vi "PointStep_Control.vi"(8 "error in (no error)":errorcluster, 9 "Temp and Field Range in":T1, 10 "ACK Q":refnum<queue>, 11 "Queue in":refnum<queue>) -> (0 "error out":errorcluster, 2 "Temp and Field Range out":T1, 3 "Queue out":refnum<queue>)   [LabVIEW 2025]
uses:
  CTLS/Sweeper.ctl
  CTLS/ACK.ctl
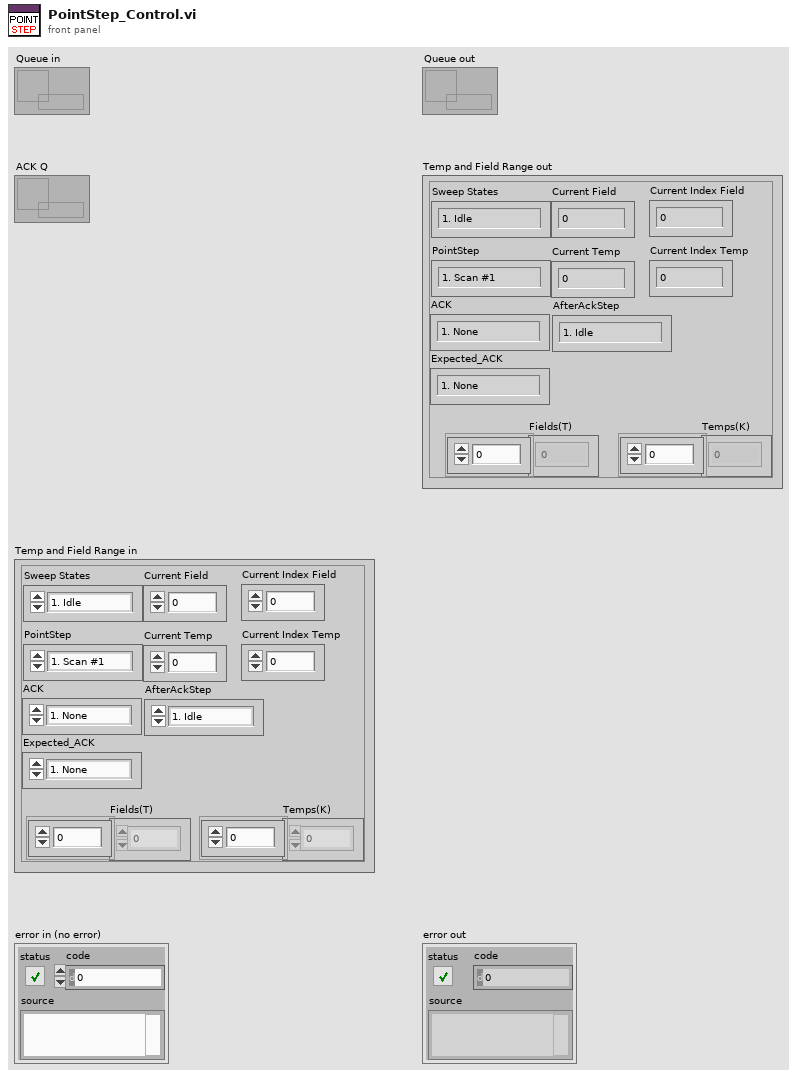
[diagram p1: front panel]
types:
  T1 = typedef "Sweeper.ctl" = cluster{"Temps(K)":dbl[], "Fields(T)":dbl[], "Sweep States":enum16{"1. Idle", "2. Start", "3. Apply_Config", "4. Run_Point_Step", "5. Wait ACK", "6. Next Field", "6. Next Temp", "8. Stop"}, "PointStep":enum16{"1. Scan #1", "2. Drift Correct (SF) #1", "3. Drift Correct (BS) #1", "4. Bias", "5. Scan #2", "6. Drift Correct (SF) #2", "7. Drift Correct (BS) #2", "8. Done"}, "Current Field":dbl, "Current Temp":dbl, "Expected_ACK":enum16{"1. None", "2. TempStable", "3. FieldStable", "4. ConfigApplied", "5. ScanDone", "6. BiasDone", "7. DriftDone (SF)", "8. DrifDone (BS)", "9. Done"}, "ACK":enum16{"1. None", "2. TempStable", "3. FieldStable", "4. ConfigApplied", "5. ScanDone", "6. BiasDone", "7. DriftDone (SF)", "8. DrifDone (BS)", "9. Done"}, "AfterAckStep":enum16{"1. Idle", "2. Start", "3. Apply_Config", "4. Run_Point_Step", "5. Wait ACK", "6. Next Field", "6. Next Temp", "8. Stop"}, "Current Index Field":i32, "Current Index Temp":i32}
  T2 = typedef "ACK.ctl" = cluster{"ACK":enum16{"1. None", "2. TempStable", "3. FieldStable", "4. ConfigApplied", "5. ScanDone", "6. BiasDone", "7. DriftDone (SF)", "8. DrifDone (BS)"}}
  T3 = enum16{"1. None", "2. TempStable", "3. FieldStable", "4. ConfigApplied", "5. ScanDone", "6. BiasDone", "7. DriftDone (SF)", "8. DrifDone (BS)", "9. Done"}
  T4 = enum16{"1. None", "2. TempStable", "3. FieldStable", "4. ConfigApplied", "5. ScanDone", "6. BiasDone", "7. DriftDone (SF)", "8. DrifDone (BS)"}
  T5 = enum16{"1. Idle", "2. Start", "3. Apply_Config", "4. Run_Point_Step", "5. Wait ACK", "6. Next Field", "6. Next Temp", "8. Stop"}
  T6 = enum16{"1. Scan #1", "2. Drift Correct (SF) #1", "3. Drift Correct (BS) #1", "4. Bias", "5. Scan #2", "6. Drift Correct (SF) #2", "7. Drift Correct (BS) #2", "8. Done"}
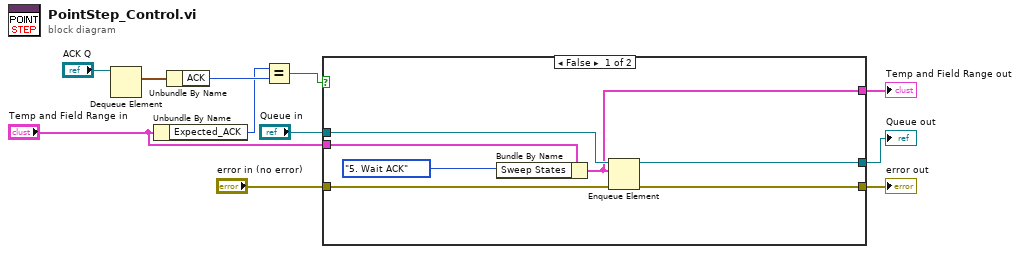
[diagram p0: block diagram]
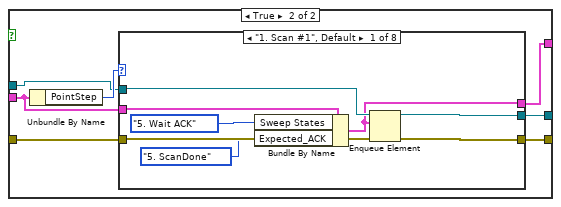
[diagram p2: hidden frame]
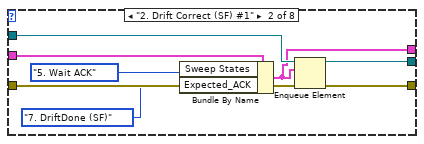
[diagram p3: hidden frame]
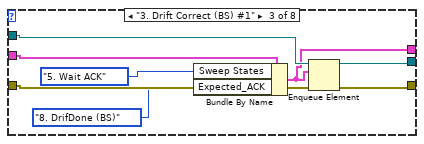
[diagram p4: hidden frame]
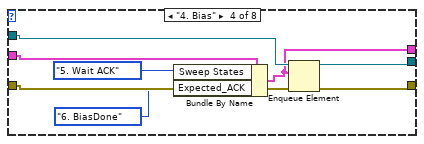
[diagram p5: hidden frame]
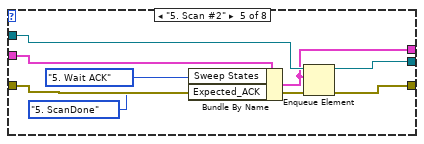
[diagram p6: hidden frame]
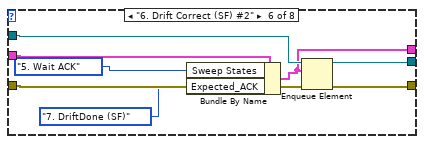
[diagram p7: hidden frame]
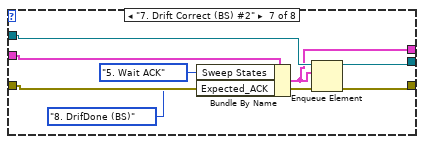
[diagram p8: hidden frame]
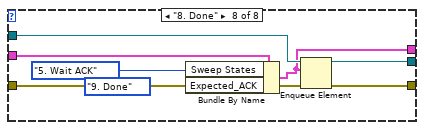
[diagram p9: hidden frame]
diagram:
  n1 = Dequeue Element(queue="ACK Q") -> (element=w2:T2)  [unwired: 2 in, 3 out]
  n2 = Unbundle By Name("Temp and Field Range in") -> ("Expected_ACK"=w3:T3)
  n3 = Unbundle By Name(w2) -> ("ACK"=w4:T4)
  n4 = Equal?(x=w3, y=w4) -> (x = y?=w5:bool)
  n5 = case shown="False" w5 {
    tunnel: "Queue in" -> [w18 w24]
    tunnel: "Temp and Field Range in" -> [w17 w23]
    tunnel: [w16 w22] -> w8
    tunnel: [w15 w21] -> w9
    tunnel: "error in (no error)" -> [w14 w20]
    tunnel: [w13 w19] -> w11
    frame False {
      n6 = Bundle By Name(cluster=w17, "Sweep States"=T5."5. Wait ACK") -> (w13:T1)
      n7 = Enqueue Element(queue=w18, element=w13, error in (no error)=w14) -> (queue out=w16:refnum<queue>, error out=w15:errorcluster)  [unwired: 1 in, 1 out]
    }
    frame True {
      n8 = Unbundle By Name(w23) -> ("PointStep"=w25:T6)
      n9 = case shown="\"1. Scan #1\", Default" w25 {
        tunnel: w24 -> [w33 w41 w49 w57 w65 w73 w81 w89]
        tunnel: w23 -> [w32 w40 w48 w56 w64 w72 w80 w88]
        tunnel: [w31 w38 w46 w54 w62 w70 w78 w86] -> w22
        tunnel: [w30 w37 w45 w53 w61 w68 w77 w85] -> w21
        tunnel: w20 -> [w29 w39 w47 w55 w63 w71 w79 w87]
        tunnel: [w28 w36 w44 w52 w60 w69 w76 w84] -> w19
        frame "1. Scan #1", Default {
          n10 = Bundle By Name(cluster=w32, "Sweep States"=T5."5. Wait ACK", "Expected_ACK"=T3."5. ScanDone") -> (w28:T1)
          n11 = Enqueue Element(queue=w33, element=w28, error in (no error)=w29) -> (queue out=w31:refnum<queue>, error out=w30:errorcluster)  [unwired: 1 in, 1 out]
        }
        frame "2. Drift Correct (SF) #1" {
          n12 = Bundle By Name(cluster=w40, "Sweep States"=T5."5. Wait ACK", "Expected_ACK"=T3."7. DriftDone (SF)") -> (w36:T1)
          n13 = Enqueue Element(queue=w41, element=w36, error in (no error)=w39) -> (queue out=w38:refnum<queue>, error out=w37:errorcluster)  [unwired: 1 in, 1 out]
        }
        frame "3. Drift Correct (BS) #1" {
          n14 = Bundle By Name(cluster=w48, "Sweep States"=T5."5. Wait ACK", "Expected_ACK"=T3."8. DrifDone (BS)") -> (w44:T1)
          n15 = Enqueue Element(queue=w49, element=w44, error in (no error)=w47) -> (queue out=w46:refnum<queue>, error out=w45:errorcluster)  [unwired: 1 in, 1 out]
        }
        frame "4. Bias" {
          n16 = Bundle By Name(cluster=w56, "Sweep States"=T5."5. Wait ACK", "Expected_ACK"=T3."6. BiasDone") -> (w52:T1)
          n17 = Enqueue Element(queue=w57, element=w52, error in (no error)=w55) -> (queue out=w54:refnum<queue>, error out=w53:errorcluster)  [unwired: 1 in, 1 out]
        }
        frame "5. Scan #2" {
          n18 = Bundle By Name(cluster=w64, "Sweep States"=T5."5. Wait ACK", "Expected_ACK"=T3."5. ScanDone") -> (w60:T1)
          n19 = Enqueue Element(queue=w65, element=w60, error in (no error)=w63) -> (queue out=w62:refnum<queue>, error out=w61:errorcluster)  [unwired: 1 in, 1 out]
        }
        frame "6. Drift Correct (SF) #2" {
          n20 = Bundle By Name(cluster=w72, "Sweep States"=T5."5. Wait ACK", "Expected_ACK"=T3."7. DriftDone (SF)") -> (w69:T1)
          n21 = Enqueue Element(queue=w73, element=w69, error in (no error)=w71) -> (queue out=w70:refnum<queue>, error out=w68:errorcluster)  [unwired: 1 in, 1 out]
        }
        frame "7. Drift Correct (BS) #2" {
          n22 = Bundle By Name(cluster=w80, "Sweep States"=T5."5. Wait ACK", "Expected_ACK"=T3."8. DrifDone (BS)") -> (w76:T1)
          n23 = Enqueue Element(queue=w81, element=w76, error in (no error)=w79) -> (queue out=w78:refnum<queue>, error out=w77:errorcluster)  [unwired: 1 in, 1 out]
        }
        frame "8. Done" {
          n24 = Bundle By Name(cluster=w88, "Sweep States"=T5."5. Wait ACK", "Expected_ACK"=T3."9. Done") -> (w84:T1)
          n25 = Enqueue Element(queue=w89, element=w84, error in (no error)=w87) -> (queue out=w86:refnum<queue>, error out=w85:errorcluster)  [unwired: 1 in, 1 out]
        }
      }
    }
  }
  "Temp and Field Range out" <- w11
  "error out" <- w9
  "Queue out" <- w8
